vi "PH_gentec_P-Link.Action check connection.vi"(0 "i ref in":refnum<vi>, 5 "error in":errorcluster) -> (14 "i ref out":refnum<vi>, 19 "error out":errorcluster)   [LabVIEW 2014, in "PH_gentec_P-Link.lvlib"]
uses:
  PH_gentec_P-Link.lvlib
  PH_Basics/PH_Powermeter_BaseClass/PH_Powermeter_BaseClass.State.ctl
  PH_Basics/PH_Powermeter_BaseClass/PH_Powermeter_BaseClass.lvlib
  instr.lib/Gentec-P-Link/gentec-P-Link - Driver.lvlib
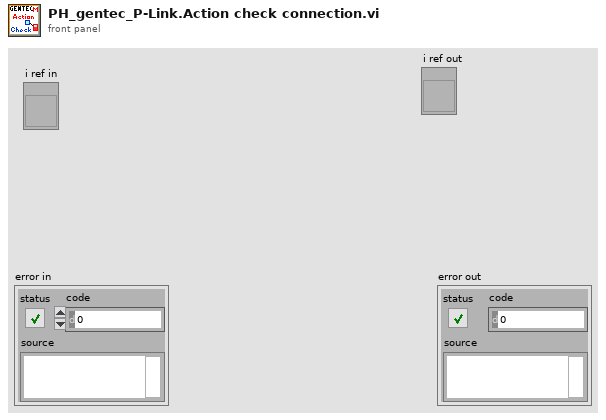
[diagram p1: front panel]
types:
  T1 = typedef "PH_Powermeter_BaseClass.lvlib/PH_Powermeter_BaseClass.State.ctl" = enum32{"off", "operating", "opened", "checked", "connected", "Sets to change", "running"}
  T2 = typedef "PH_Powermeter_BaseClass.lvlib/PH_Powermeter_BaseClass.i attribute.ctl" = cluster{"GUI References":T3, "Connection":T4, "Head Attributes":T5, "VISA resource":refnum<visa-resource-name>, "Energy":T6, "Service ID Energy":i32, "Wanted Settings":T7, "Current Settings":T7}
  T3 = typedef "PH_Powermeter_BaseClass.lvlib/PH_Powermeter_BaseClass.GUI Refs.ctl" = cluster{"Head Attributes":refnum<vi>, "Energy":refnum<vi>, "Connection":refnum<vi>, "VISA Resource":refnum<vi>, "Energy evolution":refnum<vi>, "Scaling Factor":refnum<vi>, "Range":refnum<vi>, "Wavelength":refnum<vi>, "Trigger Level":refnum<vi>, "Wanted Settings":refnum<vi>, "Current Settings":refnum<vi>}
  T4 = typedef "PH_Powermeter_BaseClass.lvlib/PH_Powermeter_BaseClass.Connection.ctl" = cluster{"failed checks":i8, "Timeout":bool, "Data read":string, "Failure":bool, "Error":bool, "State":T1}
  T5 = typedef "PH_Powermeter_BaseClass.lvlib/PH_Powermeter_BaseClass.Head Attributes.ctl" = cluster{"Instrument Type":string, "Head Version":string, "Head Name":string, "Serial Number":string, "Firmware":string, "Sensor Type":string, "MinimumRange":u32, "Maximum Range":u32, "Min Wavelength":i32, "Max Wavelength":i32}
  T6 = typedef "PH_Powermeter_BaseClass.lvlib/PH_Powermeter_BaseClass.Energy.ctl" = cluster{"current Value":dbl, "unscaled":dbl, "Scaling Factor":dbl}
  T7 = typedef "PH_Powermeter_BaseClass.lvlib/PH_gentec_BaseClass.Head Settings.ctl" = cluster{"Trigger Level":dbl, "Wavelength":u32, "Range":u32}
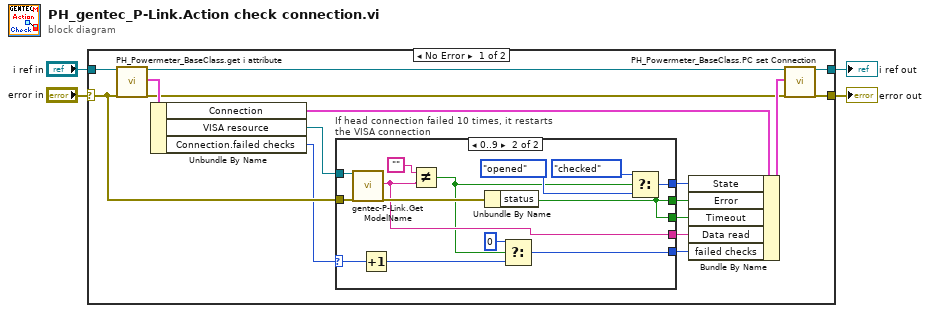
[diagram p0: block diagram]
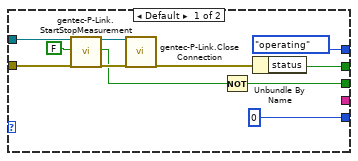
[diagram p2: hidden frame]
diagram:
  n1 = case shown="No Error" "error in" {
    selector: "error in" -> [w15 w47]
    tunnel: "i ref in" -> [w12 w46]
    tunnel: [w8 w46] -> w1
    tunnel: [w7 w47] -> w2
    frame No Error {
      n2 = call "PH_Powermeter_BaseClass.get i attribute.vi"("i ref in"=w12, "error in (no error)"=w15) -> ("i ref out"=w9:refnum<vi>, "i attribute"=w14:T2, "error out"=w6:errorcluster)  [unwired: 15 in]
      n3 = Unbundle By Name(w14) -> ("Connection"=w5:T4, "VISA resource"=w13:refnum<visa-resource-name>, "Connection.failed checks"=w11:i8)
      n4 = case "If head connection failed 10 times, it restarts the VISA connection" shown="0..9" w11 {
        selector: w11 -> [_ w43]
        tunnel: w13 -> [w25 w38]
        tunnel: w15 -> [w24 w37]
        tunnel: [w29 w32] -> w17
        tunnel: [w22 w32] -> w18
        tunnel: [_ w35] -> w19
        tunnel: [i8 0 ("Connection.failed checks") w42] -> w20
        tunnel: [PH_Powermeter_BaseClass.State."operating" ("State") w40] -> w16
        frame Default {
          n5 = call "gentec-P-Link.StartStopMeasurement.vi"("VISA resource name"=w25, "Start/Stop"=FALSE, "error in (no error)"=w24) -> ("VISA resource name"=w27:refnum<visa-resource-name>, "Sucess?"=w21:bool, "error out"=w26:errorcluster)  [unwired: 13 in, 1 out]
          n6 = call "gentec-P-Link.Close Connection.vi"("VISA resource name"=w27, "error in (no error)"=w26) -> ("error out"=w23:errorcluster)  [unwired: 17 in]
          n7 = Not(x=w21) -> (.not. x?=w22:bool)
          n8 = Unbundle By Name(w23) -> ("status"=w29:bool)
        }
        frame 0..9 {
          n9 = call "gentec-P-Link.Get ModelName.vi"("VISA resource name"=w38, "error in (no error)"=w37) -> ("Head-ModelName"=w35:string, "error out"=w36:errorcluster)  [unwired: 15 in, 1 out]
          n10 = Increment(x=w43) -> (x+1=w45:i8)
          n11 = Not Equal?(x="", y=w35) -> (x != y?=w33:bool)
          n12 = Unbundle By Name(w36) -> ("status"=w32:bool)
          n13 = Select(t=i8 0, s=w33, f=w45) -> (s? t:f=w42:i8)
          n14 = Select(t=PH_Powermeter_BaseClass.State."checked" ("State"), s=w33, f=PH_Powermeter_BaseClass.State."opened" ("State")) -> (s? t:f=w40:T1)
        }
      }
      n15 = Bundle By Name(cluster=w5, "State"=w16, "Error"=w17, "Timeout"=w18, "Data read"=w19, "failed checks"=w20) -> (w10:T4)
      n16 = call "PH_Powermeter_BaseClass.PC set Connection.vi"("VI in"=w9, "Connection"=w10, "error in (no error)"=w6) -> ("VI out"=w8:refnum<vi>, "error out"=w7:errorcluster)  [unwired: 15 in]
    }
    frame Error {
    }
  }
  "error out" <- w2
  "i ref out" <- w1
